vi "solar_voy_def Export (Interface_LINC).vi"(10 "LINC_INTERFACE":T2={"name"="", "hostname"="localhost", "port"=0, "handshake_enabled"=TRUE, "response_timeout"=30.0, "read_timeout"=nan, "write_timeout"=30.0, "length_bitoffset"=0, "length_bitsize"=32, "length_value_offset"=4, "fieldname_guid"="HDR_GUID", "endianness"=enum."BIG", "fieldname_cmd_length"="HDR_LENGTH", "Targets"=[]}) -> (2 "INTERFACE":T1)   [LabVIEW 2018]
doc: "This exports the LINC interface parameters to the COSMOS interface string. Refer to: http://cosmosrb.com/docs/interfaces/"
uses:
  solar_voy_def_ctl INTERFACE.ctl
  solar_voy_def_ctl INTERFACE (LINC).ctl
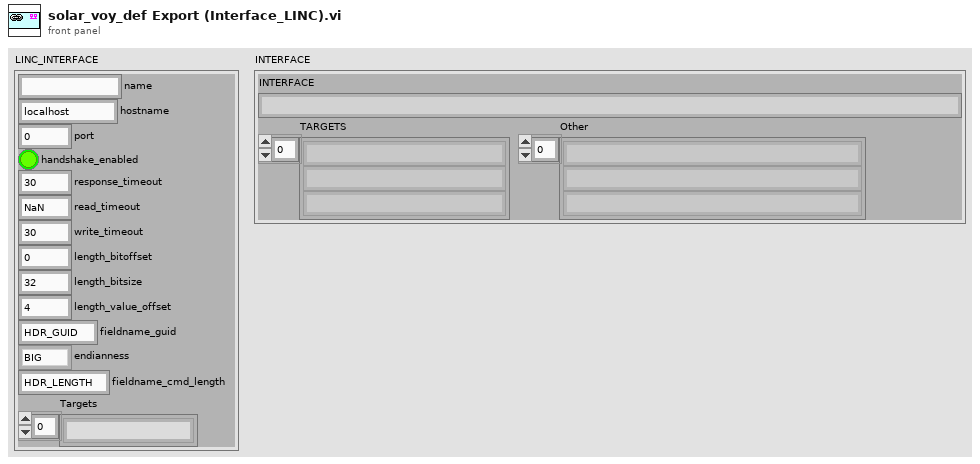
[diagram p1: front panel]
types:
  T1 = typedef "solar_voy_def_ctl INTERFACE.ctl" = cluster{"INTERFACE":string, "TARGETS":string[], "Other":string[]}
  T2 = typedef "solar_voy_def_ctl INTERFACE (LINC).ctl" = cluster{"name":string, "hostname":string, "port":u16, "handshake_enabled":bool, "response_timeout":dbl, "read_timeout":dbl, "write_timeout":dbl, "length_bitoffset":i32, "length_bitsize":i32, "length_value_offset":i32, "fieldname_guid":string, "endianness":enum8{"BIG", "LITTLE"}, "fieldname_cmd_length":string, "Targets":string[]}
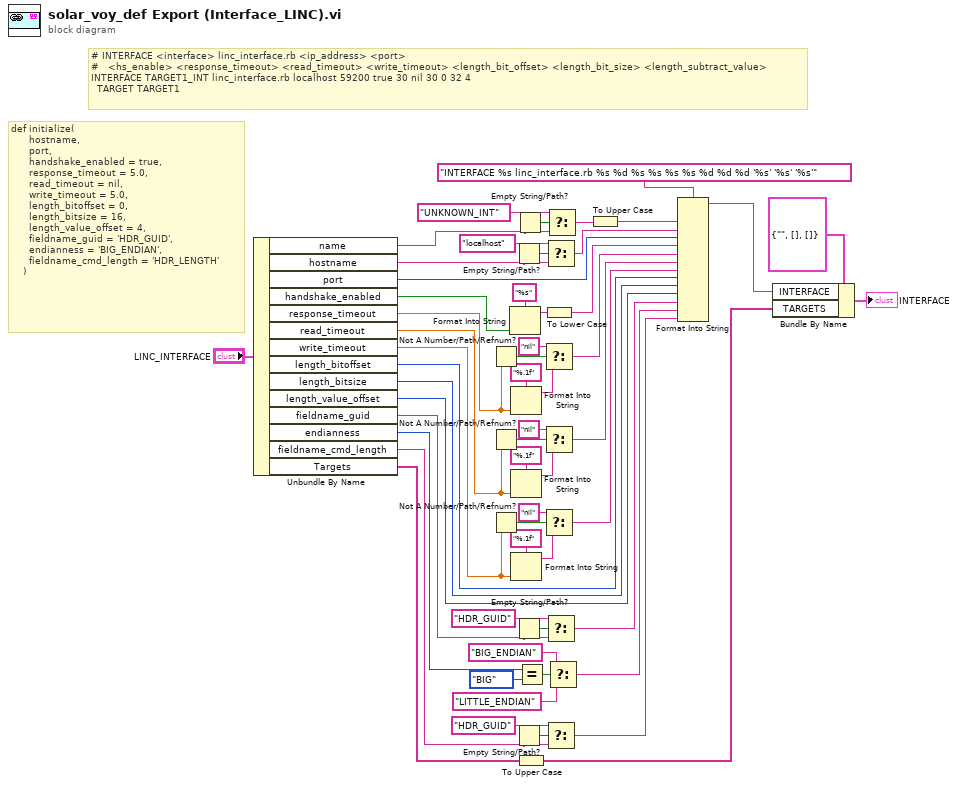
[diagram p0: block diagram]
diagram:
  # "# INTERFACE <interface> linc_interface.rb <ip_address> <port>\n#   <hs_enable> <response_timeout> <read_timeout> <write_timeout> <length_bit_offset> <length_bit_size> <length_subtract_value>\nINTERFACE TARGET1_INT linc_interface.rb localhost 59200 true 30 nil 30 0 32 4\n  TARGET TARGET1"
  # "def initialize(\n      hostname,\n      port,\n      handshake_enabled = true,\n      response_timeout = 5.0,\n      read_timeout = nil,\n      write_timeout = 5.0,\n      length_bitoffset = 0,\n      length_bitsize = 16,\n      length_value_offset = 4,\n      fieldname_guid = 'HDR_GUID',\n      endianness = 'BIG_ENDIAN',\n      fieldname_cmd_length = 'HDR_LENGTH'\n    )"
  n1 = Unbundle By Name("LINC_INTERFACE") -> ("name"=w47:string, "hostname"=w50:string, "port"=w49:u16, "handshake_enabled"=w9:bool, "response_timeout"=w41:dbl, "read_timeout"=w34:dbl, "write_timeout"=w28:dbl, "length_bitoffset"=w26:i32, "length_bitsize"=w25:i32, "length_value_offset"=w24:i32, "fieldname_guid"=w21:string, "endianness"=w19:enum8{"BIG", "LITTLE"}, "fieldname_cmd_length"=w11:string, "Targets"=w5:string[])
  n2 = Not A Number/Path/Refnum?(number/path/refnum=w41) -> (NaN/Path/Refnum?=w44:bool)
  n3 = Not A Number/Path/Refnum?(number/path/refnum=w34) -> (NaN/Path/Refnum?=w35:bool)
  n4 = Not A Number/Path/Refnum?(number/path/refnum=w28) -> (NaN/Path/Refnum?=w32:bool)
  n5 = Format Into String(format string="%s", w9) -> (resulting string=w7:string)  [unwired: 2 in, 1 out]
  n6 = Format Into String(format string="%.1f", w41) -> (resulting string=w39:string)  [unwired: 2 in, 1 out]
  n7 = Format Into String(format string="%.1f", w34) -> (resulting string=w38:string)  [unwired: 2 in, 1 out]
  n8 = Format Into String(format string="%.1f", w28) -> (resulting string=w29:string)  [unwired: 2 in, 1 out]
  n9 = Empty String/Path?(string/path=w50) -> (empty?=w55:bool)
  n10 = Empty String/Path?(string/path=w21) -> (empty?=w22:bool)
  n11 = Empty String/Path?(string/path=w11) -> (empty?=w13:bool)
  n12 = Empty String/Path?(string/path=w47) -> (empty?=w48:bool)
  n13 = To Upper Case(1:w5) -> (0:w1:string[])
  n14 = Equal?(x=w19, y=enum8{"BIG", "LITTLE"}."BIG") -> (x = y?=w17:bool)
  n15 = To Lower Case(string=w7) -> (all lower case string=w6:string)
  n16 = Select(t="nil", s=w44, f=w39) -> (s? t:f=w42:string)
  n17 = Select(t="nil", s=w35, f=w38) -> (s? t:f=w33:string)
  n18 = Select(t="nil", s=w32, f=w29) -> (s? t:f=w27:string)
  n19 = Select(t="localhost", s=w55, f=w50) -> (s? t:f=w53:string)
  n20 = Select(t="HDR_GUID", s=w22, f=w21) -> (s? t:f=w20:string)
  n21 = Select(t="HDR_GUID", s=w13, f=w11) -> (s? t:f=w10:string)
  n22 = Select(t="UNKNOWN_INT", s=w48, f=w47) -> (s? t:f=w45:string)
  n23 = Select(t="BIG_ENDIAN", s=w17, f="LITTLE_ENDIAN" ("t")) -> (s? t:f=w14:string)
  n24 = To Upper Case(1:w45) -> (0:w52:string)
  n25 = Format Into String(format string="INTERFACE %s linc_interface.rb %s %d %s %s %s %s %d %d %d '%s' '%s' '%s'" ("Definitions"), w52, w53, w49, w6, w42, w33, w27, w26, w25, w24, w20, w14, w10) -> (resulting string=w2:string)  [unwired: 2 in, 1 out]
  n26 = Bundle By Name(cluster=T1 {"INTERFACE"="", "TARGETS"=[], "Other"=[]} ("INTERFACE"), "INTERFACE"=w2, "TARGETS"=w1) -> (→"INTERFACE":T1)
